vi "Motion_xbee_3Radars.vi"(0 "VISA resource name":refnum<visa-resource-name>="COM1", 1 "baud rate":u32=9600, 4 "data bits":u16=8 min=5 max=8 step=1, 5 "parity":u16(ring) items=["None", "Odd", "Even", "Mark", "Space"], 7 "stop bits":u16=10, 9 "XON Character":u8=17 format="%.0x", 14 "XOFF Character":u8=19 format="%.0x", 15 "timeout (ms)":u32=10000, 21 "End read on termination character?":bool, 24 "termination char\n(0xA = '\\n' = LF)":u8=10 format="%.0x", 25 "buffer size":u32=4096) -> ()   [LabVIEW 2015]
doc: "The Advanced Serial Read and Write example performs a Serial Port Read, a Serial Port Write, or a combination of these actions while setting some advanced serial features like buffer size, termination characters, and XON/XOFF flow control. The user selects the actions (read or write) on the front panel. If both are selected, the VI will write the data first, read the data and then close the VISA session that is opened to the port. \n\nThe parameters set for the serial port must match the parameters of the connected instrument or device. In this example, the bytes to read parameter specifies the number of bytes that the serial port reads. If there were more bytes at the port than the number specified in bytes to read, those bytes would not be read. Also, if you specify to read more bytes than the number of bytes actually read, you might receive a timeout error message.\n\nINSTRUCTIONS:\n1) Select the serial resource and configuration parameters (baud rate, data bits, parity, stop bits, flow control).\n2) Termination character can be enabled and set. Also, set the required input buffer size prior to running the example.\n3) Select the operations to be performed. \n4) Connect the serial port to your device. If no device is available, perform a loopback test by doing one of the following. Short pins 2 and 3 on a RS-232 cable or short pin 4 to pin 8 and pin 5 to pin 9 on a RS-485/422 cable. \n5) Run the VI to see the data read. (The \"read string\" will match the \"string to write\" if a loopback test was performed.)\n\nThis example exposes several advanced features that you may need for your application. Not all applications need all the features shown in this example. The input buffer size is likely an important setting that you want to control in your application. This example expands upon the flow control option for XON and XOFF, allowing the user to choose those control characters. The timeout parameter has been brought to the front panel so a user can specify the time period the VISA Read will wait for the number of bytes to read before timing out. Also, the user has several controls for the termination character, which is discussed later.\n\nNote that you can press the write and read buttons and change the bytes to read parameters on the fly, while the example is running. However, you must stop the example to change the other configuration parameters after the example has started running, and then run again.\n\nSet the I/O buffer size slightly higher the amount of data you expect to receive. This is very important for applications that don't use flow control, as you may lose characters if the receive buffer overflows.\n\nSetting the timeout period ensures that the operation returns with a timeout error if the operation cannot be performed in the specified time period. \n\nSome devices require a termination character in order to identify the end of command strings. Some devices send a termination character to signify the end of data to be read. \n\nThis example shows how you can end the Read operation once a termination character is detected in the buffer and/or append a termination character at the end of the Write data. To enable the Read to end on a termination character, use the VISA Configure Serial Port or use the VISA Properties Serial End Mode for Reads, Termination Character Enable, and Termination Character. To end the Write with a termination character, use the VISA Properties Serial End Mode for Writes, the Send End Enable, and Termination Character. In this example, the same termination character is used for both the Read and the Write. You can specify two different characters for your application, if desired.\n\nYour application may require specific characters for the XON/XOFF Flow Control. You can specify these characters with the VISA Properties Flow Control XOFF Character and Flow Control XON Character. Note that if the standard XON and XOFF characters are used, then decimal 17 and 19 are unavailable for data values. Remember that using flow control and setting an adequate buffer size allow you to prevent buffer overflows."
uses:
  <vilib>/Instr/_visa.llb/VISA Configure Serial Port (Instr).vi
panel:
  out "I/Q":dynamicdata(graph)
  out "Spectrum":waveform(dbl)(graph)
  out "I/Q":dynamicdata(graph)
  out "Spectrum":waveform(dbl)(graph)
  out "Spectrum":waveform(dbl)(graph)
  out "I/Q channels":dynamicdata(graph)
  in  "Data saving path":path=path "C:/Users/zpeng/OneDrive - Texas Tech University/Desktop/BeamSteering/data"
  in  "Save raw data":bool
  in  "FFT":i32=800
  in  "flow control":u16(ring) items=["None"=0, "XON/XOFF"=1, "RTS/CTS"=2, "DTR/DSR"=4]
  # "Radar 2"
  # "Radar 3"
  # "Radar 1"
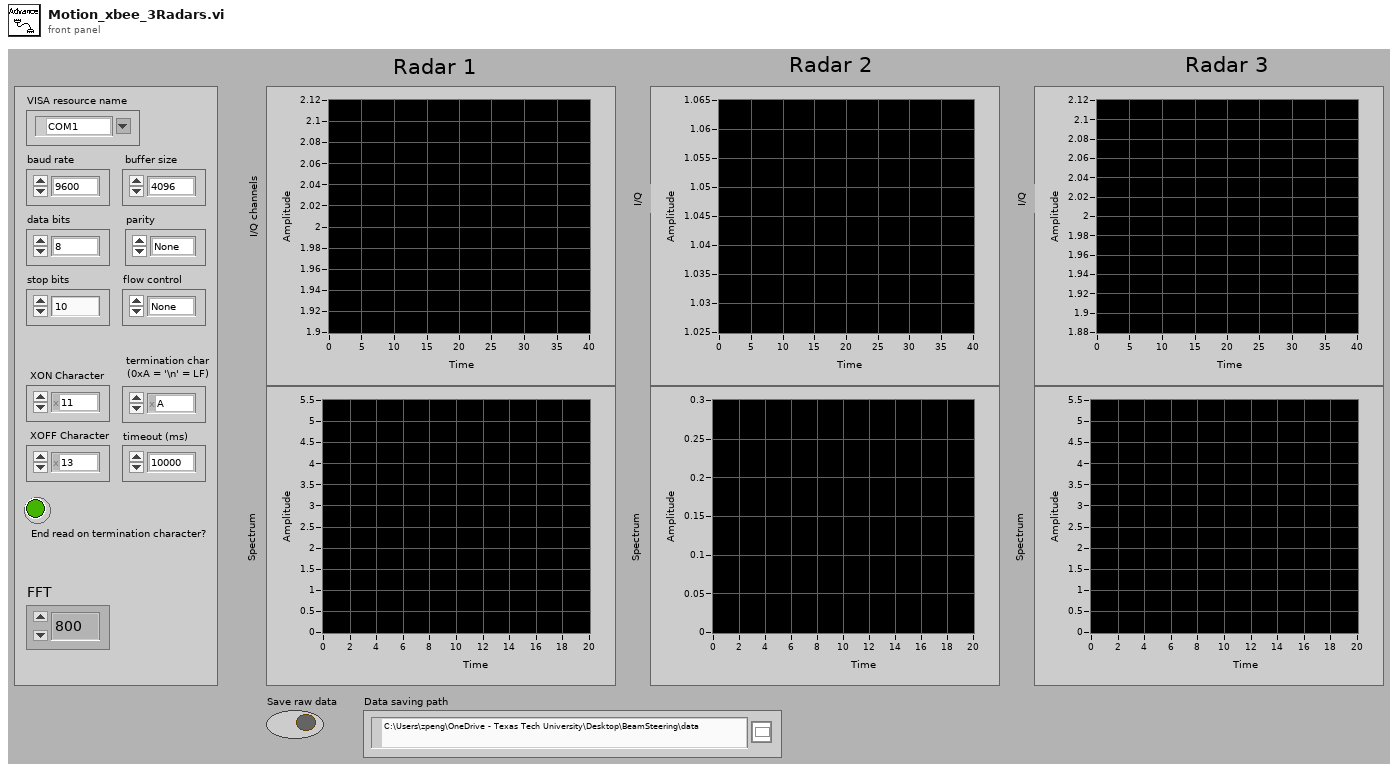
[diagram p1: front panel]
types:
  T1 = cluster{"VISA resource name out":refnum<visa-resource-name>, "error IO":errorcluster, "y":u8, i32, "Data saving path":path, "Save raw data":bool}
  T2 = cluster{"VISA resource out ":refnum<visa-resource-name>, "error out":errorcluster, "y":u8, i32, "Data saving path":path, "Save raw data":bool}
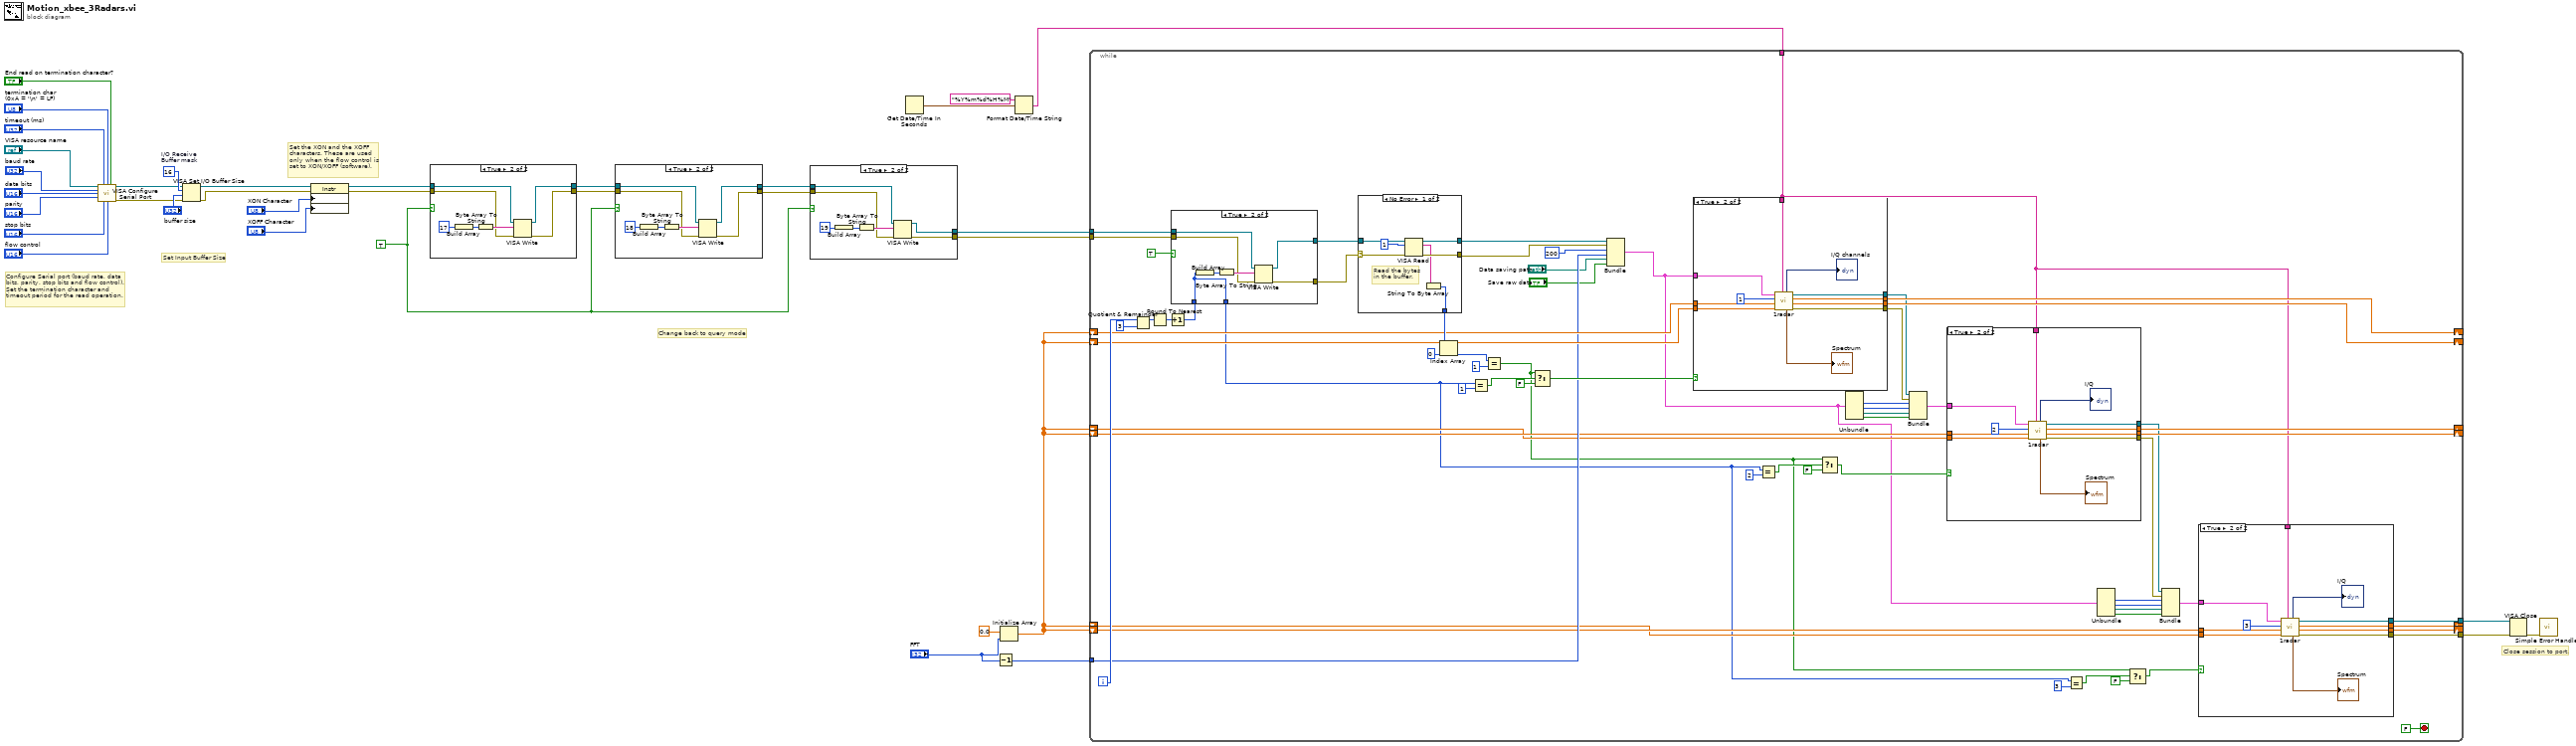
[diagram p0: block diagram]
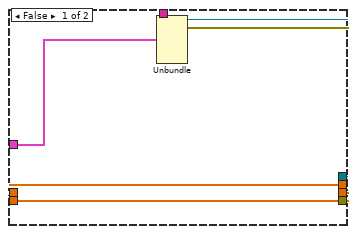
[diagram p5: hidden frame]
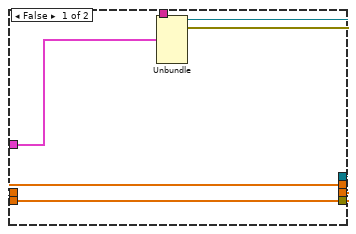
[diagram p6: hidden frame]
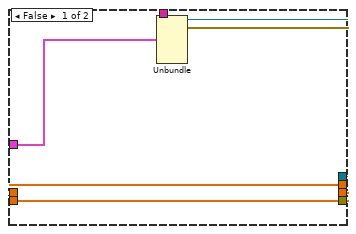
[diagram p8: hidden frame]
diagram:
  w3 = TRUE
  w29 = u16 16  # I/O Receive Buffer mask
  # "Change back to query mode"
  # "Set the XON and the XOFF\ncharacters. These are used\nonly when the flow control is\nset to XON/XOFF (software)."
  # "Configure Serial port (baud rate, data\nbits, parity, stop bits and flow control).\nSet the termination character and\ntimeout period for the read operation."
  # "Set Input Buffer Size"
  # "Close session to port."
  n1 = call-poly "VISA Configure Serial Port"("VISA resource name"="VISA resource name", "timeout (10sec)"="timeout (ms)", "termination char\n(0xA = '\\n' = LF)"="termination char\n(0xA = '\\n' = LF)", "Enable Termination\nChar (T)"="End read on termination character?", "baud rate (9600)"="baud rate", "data bits (8)"="data bits", "parity (0:none)"="parity", "stop bits (10: 1 bit)"="stop bits", "flow control (0:none)"="flow control") -> ("VISA resource name out"=w15:refnum<visa-resource-name>, "error out"=w14:errorcluster)  [unwired: 1 in, 4 out]
  n2 = VISA Set I/O Buffer Size(VISA resource name=w15, mask (16)=w29, size (4096)="buffer size", error in (no error)=w14) -> (VISA resource name out=w25:refnum<visa-resource-name>, error out=w24:errorcluster)
  n3 = property class="Instr"(reference=w25, error in=w24, "Serial Settings:Flow Control XON Character"="XON Character", "Serial Settings:Flow Control XOFF Character"="XOFF Character") -> (reference out=w9:refnum<visa-resource-name>, error out=w8:errorcluster)
  n4 = case shown="True" w3 {
    tunnel: w8 -> [w38 w44]
    tunnel: w9 -> [w37 w43]
    tunnel: [w37 w42] -> w7
    tunnel: [w38 w41] -> w6
    frame False {
    }
    frame True {
      n5 = Build Array(u8 17 ("element")) -> (w40:u8[])
      n6 = Byte Array To String(unsigned byte array=w40) -> (string=w45:string)
      n7 = VISA Write(VISA resource name=w43, write buffer=w45, error in (no error)=w44) -> (VISA resource name out=w42:refnum<visa-resource-name>, error out=w41:errorcluster)  [unwired: 1 out]
    }
  }
  n8 = case shown="True" w3 {
    tunnel: w6 -> [w47 w53]
    tunnel: w7 -> [w46 w52]
    tunnel: [w46 w51] -> w5
    tunnel: [w47 w50] -> w4
    frame False {
    }
    frame True {
      n9 = Build Array(u8 18 ("element")) -> (w49:u8[])
      n10 = Byte Array To String(unsigned byte array=w49) -> (string=w54:string)
      n11 = VISA Write(VISA resource name=w52, write buffer=w54, error in (no error)=w53) -> (VISA resource name out=w51:refnum<visa-resource-name>, error out=w50:errorcluster)  [unwired: 1 out]
    }
  }
  n12 = case shown="True" w3 {
    tunnel: w4 -> [w56 w62]
    tunnel: w5 -> [w55 w61]
    tunnel: [w55 w60] -> w1
    tunnel: [w56 w59] -> w2
    frame False {
    }
    frame True {
      n13 = Build Array(u8 19 ("element")) -> (w58:u8[])
      n14 = Byte Array To String(unsigned byte array=w58) -> (string=w63:string)
      n15 = VISA Write(VISA resource name=w61, write buffer=w63, error in (no error)=w62) -> (VISA resource name out=w60:refnum<visa-resource-name>, error out=w59:errorcluster)  [unwired: 1 out]
    }
  }
  n16 = Get Date/Time In Seconds() -> (seconds since 1Jan1904=w12:timestamp)
  n17 = Decrement(x="FFT") -> (x-1=w18:i32)
  n18 = Initialize Array(0.0 ("element"), "FFT") -> (w10:dbl[])
  n19 = Format Date/Time String(time format string (%c)="%Y%m%d%H%M", seconds (now)=w12) -> (date/time string=w11:string)  [unwired: 1 in]
  n20 = while {
    tunnel: w18 -> [w103]
    tunnel: w1 -> [w64]
    tunnel: [w66] -> w20
    tunnel: w2 -> [w125]
    tunnel: [w65] -> w19
    shift-right: [w126] -> _
    shift-left: w10 -> [w107]
    shift-right: [w127] -> _
    shift-left: w10 -> [w108]
    tunnel: w11 -> [w79]
    shift-right: [w91] -> _
    shift-left: w10 -> [w95]
    shift-right: [w90] -> _
    shift-left: w10 -> [w94]
    shift-right: [w74] -> _
    shift-left: w10 -> [w76]
    shift-right: [w73] -> _
    shift-left: w10 -> [w75]
    i -> [w117]
    stop <- FALSE stop-if-true
    n21 = Quotient & Remainder(x=w117, y=3) -> (x-y*floor(x/y)=w118:i32)  [unwired: 1 out]
    n22 = Round To Nearest(number=w118) -> (nearest integer value=w115:i32)
    n23 = Increment(x=w115) -> (x+1=w112:i32)
    n24 = case shown="True" TRUE {
      tunnel: w125 -> [w188 w194]
      tunnel: w64 -> [w187 w193]
      tunnel: [w187 w192] -> w122
      tunnel: [w188 w191] -> w123
      tunnel: w112 -> [_ w189]
      tunnel: [_ w189] -> w67
      frame False {
      }
      frame True {
        n25 = Build Array(w189) -> (w190:i32[])
        n26 = Byte Array To String(unsigned byte array=w190) -> (string=w195:string)
        n27 = VISA Write(VISA resource name=w193, write buffer=w195, error in (no error)=w194) -> (VISA resource name out=w192:refnum<visa-resource-name>, error out=w191:errorcluster)  [unwired: 1 out]
      }
    }
    n28 = case "Read bytes from port." shown="No Error" w123 {
      selector: w123 -> [w164 w169]
      tunnel: [w166 w169] -> w105
      tunnel: [w167 w170] -> w106
      tunnel: w122 -> [w165 w170]
      tunnel: [w162 u8[] [] ("unsigned byte array")] -> w121
      frame No Error {
        # "Read the bytes\nin the buffer."
        n29 = VISA Read(VISA resource name=w165, byte count=u32 1, error in (no error)=w164) -> (VISA resource name out=w167:refnum<visa-resource-name>, read buffer=w163:string, error out=w166:errorcluster)  [unwired: 1 out]
        n30 = String To Byte Array(string=w163) -> (unsigned byte array=w162:u8[])
      }
      frame Error {
        # "Error occurred \nreading Bytes at \nSerial Port"
      }
    }
    n31 = Index Array(array=w121, index=0) -> (element=w119:u8)
    n32 = Equal?(x=w67, y=1) -> (x = y?=w110:bool)
    n33 = Equal?(x=w119, y=u8 1) -> (x = y?=w68:bool)
    n34 = Select(t=w68, s=w110, f=FALSE) -> (s? t:f=w114:bool)
    n35 = Bundle("VISA resource name out"=w106, "error IO"=w105, "y"=u8 200, w103, "Data saving path"="Data saving path", "Save raw data"="Save raw data") -> (w81:T1)  [unwired: 1 in]
    n36 = case shown="True" w114 {
      tunnel: [w175 w180] -> w127
      tunnel: [w174 w179] -> w126
      tunnel: [w172 w182] -> w93
      tunnel: [w171 w181] -> w92
      tunnel: w79 -> [_ w178]
      tunnel: w108 -> [w175 w184]
      tunnel: w107 -> [w174 w183]
      tunnel: w81 -> [w173 w186]
      frame False {
        n37 = Unbundle(w173) -> ("VISA resource name out"=w172:refnum<visa-resource-name>, "error IO"=w171:errorcluster)  [unwired: 4 out]
      }
      frame True {
        n38 = call "1radar.vi"("date/time string"=w178, "Q"=w183, "I"=w184, "radar number"=u8 1 ("y"), "input cluster"=w186) -> ("error out"=w181:errorcluster, "Q out"=w179:dbl[], "I out"=w180:dbl[], "VISA resource out"=w182:refnum<visa-resource-name>, "Spectrum"=→"Spectrum":waveform(dbl), "I/Q channels"=→"I/Q channels":dynamicdata)  [unwired: 1 in]
      }
    }
    n39 = Equal?(x=w67, y=2) -> (x = y?=w89:bool)
    n40 = Select(t=w68, s=w89, f=FALSE) -> (s? t:f=w86:bool)
    n41 = Unbundle(w81) -> ("y"=w100:u8, w99:i32, "Data saving path"=w98:path, "Save raw data"=w97:bool)  [unwired: 2 out]
    n42 = Bundle("VISA resource out"=w93, "error out"=w92, "y"=w100, w99, "Data saving path"=w98, "Save raw data"=w97) -> (w96:T2)  [unwired: 1 in]
    n43 = case shown="True" w86 {
      tunnel: [w149 w154] -> w91
      tunnel: [w148 w153] -> w90
      tunnel: [w146 w156] -> w78
      tunnel: [w145 w155] -> w77
      tunnel: w79 -> [_ w152]
      tunnel: w95 -> [w149 w158]
      tunnel: w94 -> [w148 w157]
      tunnel: w96 -> [w147 w160]
      frame False {
        n44 = Unbundle(w147) -> ("VISA resource out"=w146:refnum<visa-resource-name>, "error out"=w145:errorcluster)  [unwired: 4 out]
      }
      frame True {
        n45 = call "1radar.vi"("date/time string"=w152, "Q"=w157, "I"=w158, "radar number"=u8 2 ("y"), "input cluster"=w160) -> ("error out"=w155:errorcluster, "Q out"=w153:dbl[], "I out"=w154:dbl[], "VISA resource out"=w156:refnum<visa-resource-name>, "Spectrum"=→"Spectrum":waveform(dbl), "I/Q channels"=→"I/Q":dynamicdata)  [unwired: 1 in]
      }
    }
    n46 = Equal?(x=w67, y=3) -> (x = y?=w72:bool)
    n47 = Unbundle(w81) -> ("y"=w85:u8, w84:i32, "Data saving path"=w83:path, "Save raw data"=w82:bool)  [unwired: 2 out]
    n48 = Select(t=w68, s=w72, f=FALSE) -> (s? t:f=w69:bool)
    n49 = Bundle("VISA resource out"=w78, "error out"=w77, "y"=w85, w84, "Data saving path"=w83, "Save raw data"=w82) -> (w80:T2)  [unwired: 1 in]
    n50 = case shown="True" w69 {
      tunnel: [w133 w138] -> w74
      tunnel: [w132 w137] -> w73
      tunnel: [w130 w140] -> w66
      tunnel: [w129 w139] -> w65
      tunnel: w79 -> [_ w136]
      tunnel: w76 -> [w133 w142]
      tunnel: w75 -> [w132 w141]
      tunnel: w80 -> [w131 w144]
      frame False {
        n51 = Unbundle(w131) -> ("VISA resource out"=w130:refnum<visa-resource-name>, "error out"=w129:errorcluster)  [unwired: 4 out]
      }
      frame True {
        n52 = call "1radar.vi"("date/time string"=w136, "Q"=w141, "I"=w142, "radar number"=u8 3 ("y"), "input cluster"=w144) -> ("error out"=w139:errorcluster, "Q out"=w137:dbl[], "I out"=w138:dbl[], "VISA resource out"=w140:refnum<visa-resource-name>, "Spectrum"=→"Spectrum":waveform(dbl), "I/Q channels"=→"I/Q":dynamicdata)  [unwired: 1 in]
      }
    }
  }
  n53 = VISA Close(VISA resource name=w20, error in (no error)=w19) -> (error out=w34:errorcluster)
  n54 = call <vilib>:"Simple Error Handler.vi"("error in (no error)"=w34) -> ()  [unwired: 1 in, 8 out]
